vi "AsyncOptions.vi"() -> (3 "AsyncOptions":i32)   [LabVIEW 2020, in "jettl.lvlib"]
uses:
  jettl.lvlib
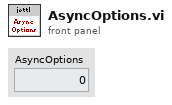
[diagram p1: front panel]
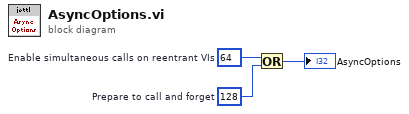
[diagram p0: block diagram]
diagram:
  w2 = 64  # Enable simultaneous calls on reentrant VIs
  w3 = 128  # Prepare to call and forget
  n1 = Or(x=w2, y=w3) -> (x .or. y?=→"AsyncOptions":i32)
